vi "Verify image path.vi"(8 "error in (no error)":errorcluster, 11 "Channel in":refnum<class "SPARC4_Channel.lvclass">) -> (0 "error out":errorcluster, 3 "Channel out":refnum<class "SPARC4_Channel.lvclass">)   [LabVIEW 2018, in "SPARC4_Channel.lvclass"]
doc: "Verify if the provided directory exists"
uses:
  SPARC4_Channel.lvclass
  SPARC4_Channel.lvclass/SPARC4_Channel.ctl
  <vilib>/Utility/error.llb/Error Cluster From Error Code.vi
  <vilib>/ErrorRing/Error Ring.xnode
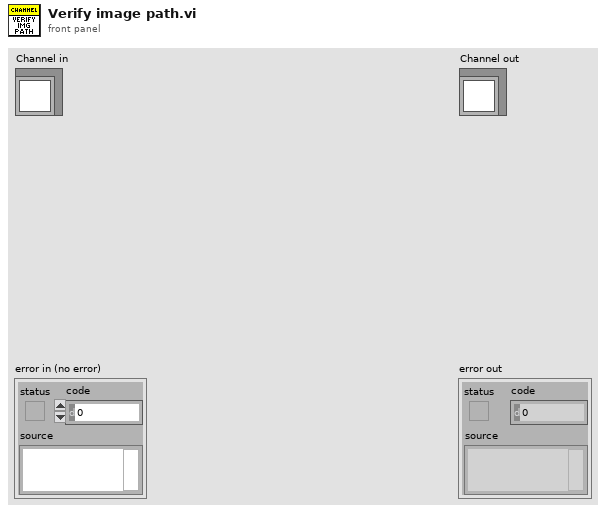
[diagram p1: front panel]
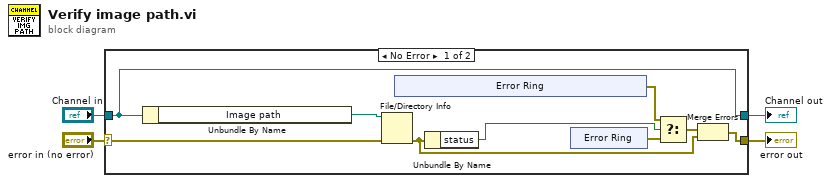
[diagram p0: block diagram]
diagram:
  n1 = case shown="No Error" "error in (no error)" {
    selector: "error in (no error)" -> [w10 w21]
    tunnel: [w11 w21] -> w3
    tunnel: [w12 w20] -> w1
    tunnel: "Channel in" -> [w12 w20]
    frame No Error {
      n2 = Unbundle By Name(w12) -> ("Image path"=w13:path)
      n3 = File/Directory Info(path=w13, error in=w10) -> (error out=w9:errorcluster)  [unwired: 6 out]
      n4 = xnode "Error Ring"() -> ("error out"=w8:errorcluster)
      n5 = Unbundle By Name(w9) -> ("status"=w6:bool)
      n6 = xnode "Error Ring"() -> ("error out"=w7:errorcluster)
      n7 = Select(t=w8, s=w6, f=w7) -> (s? t:f=w5:errorcluster)
      n8 = Merge Errors(w5, w9) -> (w11:errorcluster)
    }
    frame Error {
    }
  }
  "error out" <- w3
  "Channel out" <- w1
